vi "DCM DSI Host.vi"() -> ()   [LabVIEW 2016]
uses:
  <vilib>/addons/Software Calibration Management/XControls/SubHost.xctl
  <vilib>/Powertrain Controls/Device Drivers/DCM/Rev0/RT/System State.ctl
  <vilib>/Powertrain Controls/Device Drivers/DCM/Rev0/RT/System ADC.ctl
  <vilib>/Powertrain Controls/Device Drivers/DCM/Rev0/RT/Internal Fault.ctl
  Shared/Typedefs/System-QuickIDsArray.ctl
  <vilib>/addons/Software Calibration Management/xSCM/Controls/ID and Element.ctl
  <vilib>/Utility/miscctls.llb/LVBoundsTypeDef.ctl
  Host/Host SubVIs/VI Ref Global.vi
  <vilib>/Utility/inputDevices.llb/mouseAcquire.vi
  <vilib>/addons/Software Calibration Management/xSCM/SCM-API.lvlib
  <vilib>/Powertrain Controls/Device Drivers/DCM/Rev0/RT/DCM - RT.lvclass
  Shared/DSI-Shared.lvlib
panel:
  in  "_Subhosts":enum32{"Subhosts"}(tab)
  in  "Hidden Settings":T1(xcontrol)={"Name"="System-ExecInfo-Host (System-ExecInfo-Host)", "Host VI"=path "Host/System-ExecInfo-Host.vi", "Pairing File"=path "Host/System-ExecInfo-Host.par", "Display Name"="Execution Information"}
  in  "User Plugin (Engine)":T1(xcontrol)={"Name"="Engine-Throttle-Host (Engine-Throttle-Host)", "Host VI"=path "Host/Engine-Throttle-Host.vi", "Pairing File"=path "Host/Engine-Throttle-Host.par", "Display Name"="Throttle Control Setup"}
  in  "Engine Synchronous TTL Setup":T1(xcontrol)={"Name"="Hardware-DiffIO-Host (Hardware-DiffIO-Host)", "Host VI"=path "Host/Hardware-DiffIO-Host.vi", "Pairing File"=path "Host/Hardware-DiffIO-Host.par", "Display Name"="Differential IO Setup"}
  in  "DI Driver Bank A Setup":T1(xcontrol)={"Name"="Hardware-DI-A-Host (Hardware-DI-A-Host)", "Host VI"=path "Host/Hardware-DI-A-Host.vi", "Pairing File"=path "Host/Hardware-DI-A-Host.par", "Display Name"="DI Driver Bank A Setup"}
  in  "DCM System Setup & State":T1(xcontrol)={"Name"="Hardware-System-Host (Hardware-System-Host)", "Host VI"=path "Host/Hardware-System-Host.vi", "Pairing File"=path "Host/Hardware-System-Host.par", "Display Name"="Hardware System Setup"}
  in  "Half-H Driver Setup":T1(xcontrol)={"Name"="Hardware-HHSetup-Host (Hardware-HHSetup-Host)", "Host VI"=path "Host/Hardware-HHSetup-Host.vi", "Pairing File"=path "Host/Hardware-HHSetup-Host.par", "Display Name"="Half H Setup"}
  in  "DI Driver Bank B Setup":T1(xcontrol)={"Name"="Hardware-DI-B-Host (Hardware-DI-B-Host)", "Host VI"=path "Host/Hardware-DI-B-Host.vi", "Pairing File"=path "Host/Hardware-DI-B-Host.par", "Display Name"="DI Driver Bank B Setup"}
  in  "Differential Digital I/O Setup":T1(xcontrol)={"Name"="Hardware-DiffIO-Host (Hardware-DiffIO-Host)", "Host VI"=path "Host/Hardware-DiffIO-Host.vi", "Pairing File"=path "Host/Hardware-DiffIO-Host.par", "Display Name"="Differential IO Setup"}
  in  "Engine Position Tracking Setup":T1(xcontrol)={"Name"="Hardware-EPTx-Host (Hardware-EPTx-Host)", "Host VI"=path "Host/Hardware-EPTx-Host.vi", "Pairing File"=path "Host/Hardware-EPTx-Host.par", "Display Name"="Engine Position Tracking Setup"}
  in  "CAN Interface":T1(xcontrol)={"Name"="System-CAN-Host (System-CAN-Host)", "Host VI"=path "Host/System-CAN-Host.vi", "Pairing File"=path "Host/System-CAN-Host.par", "Display Name"="CAN Interface"}
  in  "Skip Fire Setup":T1(xcontrol)={"Name"="Hardware-Skipfire-Host (Hardware-Skipfire-Host)", "Host VI"=path "Host/Hardware-Skipfire-Host.vi", "Pairing File"=path "Host/Hardware-Skipfire-Host.par", "Display Name"="Skip Fire Setup"}
  in  "Analog Inputs Setup":T1(xcontrol)={"Name"="Engine-SystemAI-Host (Engine-SystemAI-Host)", "Host VI"=path "Host/Engine-SystemAI-Host.vi", "Pairing File"=path "Host/Engine-SystemAI-Host.par", "Display Name"="Analog Input Setup"}
  in  "DCM System ADC":T1(xcontrol)={"Name"="Hardware-System-Host (Hardware-System-Host)", "Host VI"=path "Host/Hardware-System-Host.vi", "Pairing File"=path "Host/Hardware-System-Host.par", "Display Name"="Hardware System Setup"}
  in  "DI Scope":T1(xcontrol)={"Name"="Engine-DICal-Host (Engine-DICal-Host)", "Host VI"=path "Host/Engine-DICal-Host.vi", "Pairing File"=path "Host/Engine-DICal-Host.par", "Display Name"="Injector Calibration Setup"}
  in  "HH Scope":T1(xcontrol)={"Name"="Engine-Throttle-Host (Engine-Throttle-Host)", "Host VI"=path "Host/Engine-Throttle-Host.vi", "Pairing File"=path "Host/Engine-Throttle-Host.par", "Display Name"="Throttle Control Setup"}
  in  "Plots and Tables":T1(xcontrol)={"Name"="System-ExecInfo-Host (System-ExecInfo-Host)", "Host VI"=path "Host/System-ExecInfo-Host.vi", "Pairing File"=path "Host/System-ExecInfo-Host.par", "Display Name"="Execution Information"}
  in  "Execution Information":T1(xcontrol)={"Name"="System-ExecInfo-Host (System-ExecInfo-Host)", "Host VI"=path "Host/System-ExecInfo-Host.vi", "Pairing File"=path "Host/System-ExecInfo-Host.par", "Display Name"="Execution Information"}
  in  "Channel Data":T1(xcontrol)={"Name"="Engine-SystemAI-Host (Engine-SystemAI-Host)", "Host VI"=path "Host/Engine-SystemAI-Host.vi", "Pairing File"=path "Host/Engine-SystemAI-Host.par", "Display Name"="Analog Input Setup"}
  in  "User Plugin (Asynchronous)":T1(xcontrol)={"Name"="System-User-Host (System-User-Host)", "Host VI"=path "Host/System-User-Host.vi", "Pairing File"=path "Host/System-User-Host.par", "Display Name"="System User VI"}
  in  "DI IPhase Learn":T1(xcontrol)={"Name"="Engine-RPC-Host (Engine-RPC-Host)", "Host VI"=path "Host/Engine-RPC-Host.vi", "Pairing File"=path "Host/Engine-RPC-Host.par", "Display Name"="Rail Pressure Control Setup"}
  in  "DI Control and Calibration":T1(xcontrol)={"Name"="Engine-DICal-Host (Engine-DICal-Host)", "Host VI"=path "Host/Engine-DICal-Host.vi", "Pairing File"=path "Host/Engine-DICal-Host.par", "Display Name"="Injector Calibration Setup"}
  in  "Rail Pressure Control":T1(xcontrol)={"Name"="Engine-RPC-Host (Engine-RPC-Host)", "Host VI"=path "Host/Engine-RPC-Host.vi", "Pairing File"=path "Host/Engine-RPC-Host.par", "Display Name"="Rail Pressure Control Setup"}
  in  "Electronic Throttle Control":T1(xcontrol)={"Name"="Engine-Throttle-Host (Engine-Throttle-Host)", "Host VI"=path "Host/Engine-Throttle-Host.vi", "Pairing File"=path "Host/Engine-Throttle-Host.par", "Display Name"="Throttle Control Setup"}
  in  "User Plugin (Control)":T1(xcontrol)={"Name"="Control-DIFuel-Host (Control-DIFuel-Host)", "Host VI"=path "Host/Control-DIFuel-Host.vi", "Pairing File"=path "Host/Control-DIFuel-Host.par", "Display Name"="DI Fueling Control Setup"}
  in  "Engine Fuel Control":T1(xcontrol)={"Name"="Control-DIFuel-Host (Control-DIFuel-Host)", "Host VI"=path "Host/Control-DIFuel-Host.vi", "Pairing File"=path "Host/Control-DIFuel-Host.par", "Display Name"="DI Fueling Control Setup"}
  out "_DragStart":i32
  in  "UserOS":bool
  out "_IO_Lock":bool caption="I/O Lock"
  out "Sync":bool caption="EPTx"
  in  "SyncEnable":bool
  in  "DI-B_InjectEnable":bool
  in  "DI-A_InjectEnable":bool
  in  "IO_Lock":bool
  in  "MPRD":bool
  in  "SYS|Exec|Password":string
  in  "SYS|Exec|Username":string
  in  "_Help":bool
  out "SYS|Host|Fault":bool
  in  "_AutoFit":bool
  in  "_CalTrend":bool
  in  "_CalScope":bool
  in  "_CalLoad":bool
  in  "_CalSaveAs":bool
  in  "_CalSave":bool
  in  "_RedrawList":bool
  in  "UserOSTime":sgl caption="[s]" format="%#_6p"
  out "_Battery":sgl caption="[V]"
  out "Speed":sgl caption="[RPM]"
  out "_Drive_Power":sgl caption="[V]"
  out "_ConsoleMessages":string caption="SCM Messages"
  in  "_SubHost-List":i32(listbox)=-1
  out "SYS|Exec|CalLoading":bool caption="HW"
  in  "SYS|Plot|Names":string[](array[string])
  out "SYS|Plot|Values":sgl[](array[numeric])
  in  "SYS|Plot|Units":string[](array[string])
  in  "SYS|Plot|IDs":T2
  out "_Subhost-FP.DockStates":bool[](array[boolean])
  out "_Subhost-FP.States":T4(array[ring])=[enum."Closed", enum."Closed", enum."Closed", enum."Closed", enum."Closed", enum."Closed", enum."Closed", enum."Closed", enum."Closed", enum."Closed", enum."Closed", enum."Closed", enum."Closed", enum."Closed", enum."Closed", enum."Closed", enum."Closed", enum."Closed", enum."Closed"]
  in  "_QuickValues":i32(listbox) caption="Quick Values"
  in  "SYS|Plot|Select":u8
  out "State":T5 {"System ADC"."Fan [V]" format="%#_3p"; "System ADC"."Primary B1B2 [V]" format="%#_3p"; "System ADC"."Primary B3B4 [V]" format="%#_3p"; "System ADC"."Primary A3A4 [V]" format="%#_3p"; "System ADC"."Primary A1A2 [V]" format="%#_3p"; "System ADC"."MPRD [V]" format="%#_3p"; "System ADC"."Ext HV B [V]" format="%#_3p"; "System ADC"."Ext HV A [V]" format="%#_3p"; "System ADC"."Pump Zener B [V]" format="%#_3p"; "System ADC"."Pump Zener A [V]" format="%#_3p"; "System ADC"."DI Zener B [V]" format="%#_3p"; "System ADC"."DI Zener A [V]" format="%#_3p"; "System ADC"."Key [V]" format="%#_3p"; "System ADC"."DRVP [V]" format="%#_3p"; "System ADC"."Battery [V]" format="%#_3p"; "System ADC"."FET Driver [V]" format="%#_3p"; "System ADC"."Secondary B1B2 [V]" format="%#_3p"; "System ADC"."Secondary B3B4 [V]" format="%#_3p"; "System ADC"."Secondary A3A4 [V]" format="%#_3p"; "System ADC"."Secondary A1A2 [V]" format="%#_3p"; "System ADC"."Primary Range [V]" format="%#_3p"; "System ADC"."Temp Boost B [C]" format="%#_3p"; "System ADC"."Temp Primary A [C]" format="%#_3p"; "System ADC"."Temp Secondary A [C]" format="%#_3p"; "System ADC"."Temp Fan Intake [C]" format="%#_3p"; "System ADC"."Temp CPU [C]" format="%#_3p"; "System ADC"."Temp DI Zener B [C]" format="%#_3p"; "System ADC"."Temp DI B [C]" format="%#_3p"; "System ADC"."Temp DI Zener A [C]" format="%#_3p"; "System ADC"."Temp DI A [C]" format="%#_3p"; "System ADC"."Temp HH 7-12 [C]" format="%#_3p"; "System ADC"."Temp HH 1-6 [C]" format="%#_3p"; "System ADC"."AI 12 [V]" format="%#_3p"; "System ADC"."AI 11 [V]" format="%#_3p"; "System ADC"."AI 10 [V]" format="%#_3p"; "System ADC"."AI 9 [V]" format="%#_3p"; "System ADC"."AI 8 [V]" format="%#_3p"; "System ADC"."AI 7 [V]" format="%#_3p"; "System ADC"."AI 6 [V]" format="%#_3p"; "System ADC"."AI 5 [V]" format="%#_3p"; "System ADC"."AI 4 [V]" format="%#_3p"; "System ADC"."AI 3 [V]" format="%#_3p"; "System ADC"."AI 2 [V]" format="%#_3p"; "System ADC"."AI 1 [V]" format="%#_3p"}
  # "Password"
  # "Username"
  # "One-Shot Time"
  # "Batt"
  # "Speed"
  # "DRVP"
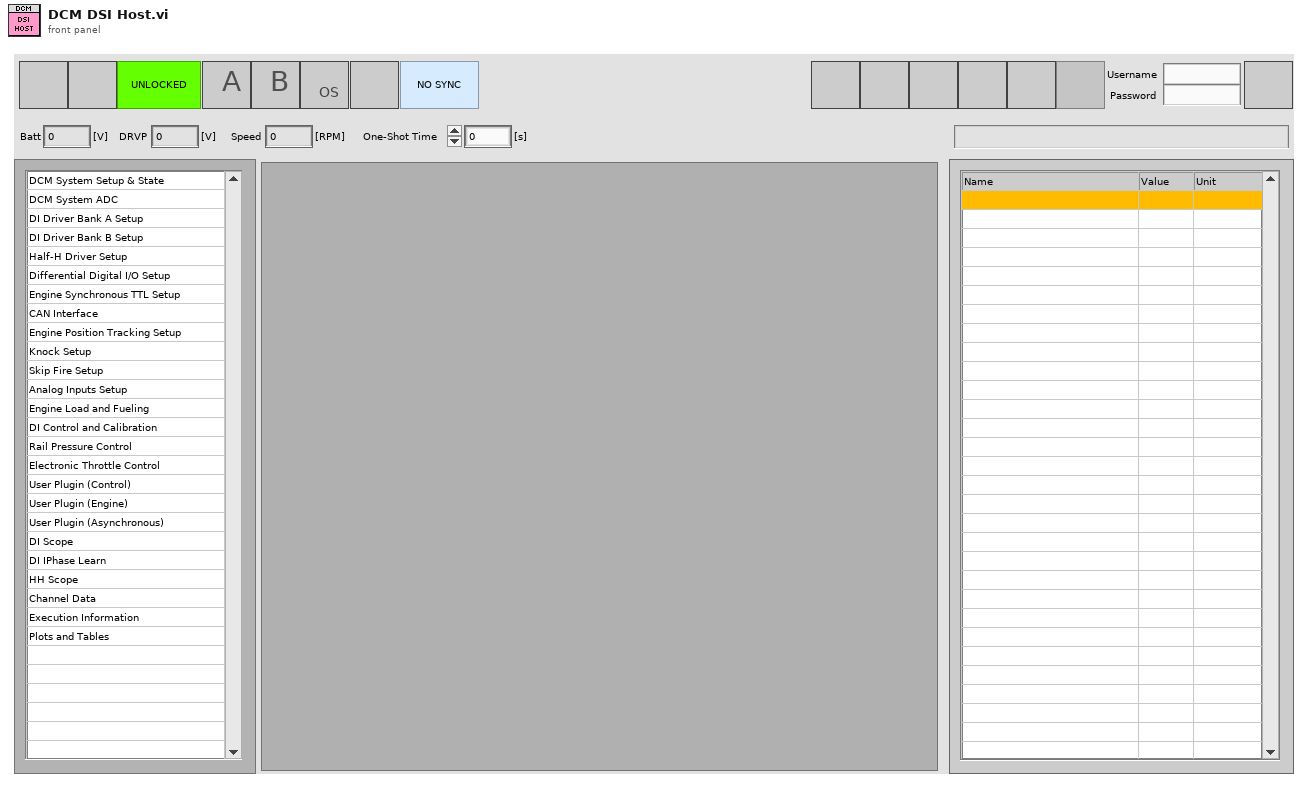
[diagram p1: front panel]
types:
  T1 = cluster{"Name":string, "Host VI":path, "Pairing File":path, "Display Name":string}
  T2 = typedef "DSI-Shared.lvlib/System-QuickIDsArray.ctl" = T3[]
  T3 = typedef "SCM-API.lvlib/ID and Element.ctl" = cluster{"ID":u32, "Element":i32[]}
  T4 = enum32{"Invalid", "Standard", "Closed", "Hidden", "Minimized", "Maximized"}[]
  T5 = typedef "DCM - RT.lvclass/System State.ctl" = cluster{"System ADC":T6, "IO Lock":bool, "HH Mode Config Error":bool, "Fan Speed 1 [RPM]":sgl, "Fan Speed 2 [RPM]":sgl, "Firmware Major Rev":u16, "Firmware Minor Rev":u16, "Internal Fault":T7, "Fault Value":dbl}
  T6 = typedef "DCM - RT.lvclass/System ADC.ctl" = cluster{"AI 1 [V]":sgl, "AI 2 [V]":sgl, "AI 3 [V]":sgl, "AI 4 [V]":sgl, "AI 5 [V]":sgl, "AI 6 [V]":sgl, "AI 7 [V]":sgl, "AI 8 [V]":sgl, "AI 9 [V]":sgl, "AI 10 [V]":sgl, "AI 11 [V]":sgl, "AI 12 [V]":sgl, "Temp HH 1-6 [C]":sgl, "Temp HH 7-12 [C]":sgl, "Temp DI A [C]":sgl, "Temp DI Zener A [C]":sgl, "Temp DI B [C]":sgl, "Temp DI Zener B [C]":sgl, "Temp CPU [C]":sgl, "Temp Fan Intake [C]":sgl, "Temp Secondary A [C]":sgl, "Temp Primary A [C]":sgl, "Temp Boost B [C]":sgl, "Primary Range [V]":sgl, "Primary A1A2 [V]":sgl, "Primary A3A4 [V]":sgl, "Primary B3B4 [V]":sgl, "Primary B1B2 [V]":sgl, "Secondary A1A2 [V]":sgl, "Secondary A3A4 [V]":sgl, "Secondary B3B4 [V]":sgl, "Secondary B1B2 [V]":sgl, "Ext HV A [V]":sgl, "Ext HV B [V]":sgl, "FET Driver [V]":sgl, "Fan [V]":sgl, "Battery [V]":sgl, "DRVP [V]":sgl, "Key [V]":sgl, "DI Zener A [V]":sgl, "DI Zener B [V]":sgl, "Pump Zener A [V]":sgl, "Pump Zener B [V]":sgl, "MPRD [V]":sgl}
  T7 = typedef "DCM - RT.lvclass/Internal Fault.ctl" = enum32{"None", "Temp HH 1-6", "Temp HH 7-12", "Temp DI A", "Temp DI Zener A", "Temp DI B", "Temp DI Zener B", "Temp Intake", "Temp Primary A", "Temp Secondary A", "Temp Boost B", "Temp CPU", "Low Battery", "Inrush Protection", "A Run Enable", "B Run Enable", "Fan Speed"}
  T8 = typedef "LVBoundsTypeDef.ctl" = cluster{"Width":u32, "Height":u32}
  T9 = enum8{"Enabled", "Disabled", "Disabled and Grayed Out"}
  T10 = enum32{"Invalid", "Standard", "Closed", "Hidden", "Minimized", "Maximized"}
  T11 = enum16{"Save Workspace", "Exit", "Stop Host Application", "Stop Target", "Set Target Time", "Fault File", "Fault Display", "Silence Alarms", "Calibration Differencer", "Save Calibration", "Save Calibration As", "Get Calibration File", "Set Calibration File", "Load Calibration File", "CalScope", "CalTrend"}
  T12 = cluster{u32, "DCM System Setup & State":cluster{"Name":string, "Host VI":path, "Pairing File":path, "Display Name":string}}
  T13 = cluster{u32, "DCM System ADC":cluster{"Name":string, "Host VI":path, "Pairing File":path, "Display Name":string}}
  T14 = cluster{u32, "DI Driver Bank A Setup":cluster{"Name":string, "Host VI":path, "Pairing File":path, "Display Name":string}}
  T15 = cluster{u32, "DI Driver Bank B Setup":cluster{"Name":string, "Host VI":path, "Pairing File":path, "Display Name":string}}
  T16 = cluster{u32, "Half-H Driver Setup":cluster{"Name":string, "Host VI":path, "Pairing File":path, "Display Name":string}}
  T17 = cluster{u32, "Differential Digital I/O Setup":cluster{"Name":string, "Host VI":path, "Pairing File":path, "Display Name":string}}
  T18 = cluster{u32, "Engine Synchronous TTL Setup":cluster{"Name":string, "Host VI":path, "Pairing File":path, "Display Name":string}}
  T19 = cluster{u32, "CAN Interface":cluster{"Name":string, "Host VI":path, "Pairing File":path, "Display Name":string}}
  T20 = cluster{u32, "Engine Position Tracking Setup":cluster{"Name":string, "Host VI":path, "Pairing File":path, "Display Name":string}}
  T21 = cluster{u32, "Skip Fire Setup":cluster{"Name":string, "Host VI":path, "Pairing File":path, "Display Name":string}}
  T22 = cluster{u32, "Analog Inputs Setup":cluster{"Name":string, "Host VI":path, "Pairing File":path, "Display Name":string}}
  T23 = cluster{u32, "Engine Fuel Control":cluster{"Name":string, "Host VI":path, "Pairing File":path, "Display Name":string}}
  T24 = cluster{u32, "DI Control and Calibration":cluster{"Name":string, "Host VI":path, "Pairing File":path, "Display Name":string}}
  T25 = cluster{u32, "Rail Pressure Control":cluster{"Name":string, "Host VI":path, "Pairing File":path, "Display Name":string}}
  T26 = cluster{u32, "Electronic Throttle Control":cluster{"Name":string, "Host VI":path, "Pairing File":path, "Display Name":string}}
  T27 = cluster{u32, "User Plugin (Control)":cluster{"Name":string, "Host VI":path, "Pairing File":path, "Display Name":string}}
  T28 = cluster{u32, "User Plugin (Engine)":cluster{"Name":string, "Host VI":path, "Pairing File":path, "Display Name":string}}
  T29 = cluster{u32, "DI Scope":cluster{"Name":string, "Host VI":path, "Pairing File":path, "Display Name":string}}
  T30 = cluster{u32, "DI IPhase Learn":cluster{"Name":string, "Host VI":path, "Pairing File":path, "Display Name":string}}
  T31 = cluster{u32, "HH Scope":cluster{"Name":string, "Host VI":path, "Pairing File":path, "Display Name":string}}
  T32 = cluster{u32, "Channel Data":cluster{"Name":string, "Host VI":path, "Pairing File":path, "Display Name":string}}
  T33 = cluster{u32, "Execution Information":cluster{"Name":string, "Host VI":path, "Pairing File":path, "Display Name":string}}
  T34 = cluster{u32, "Plots and Tables":cluster{"Name":string, "Host VI":path, "Pairing File":path, "Display Name":string}}
  T35 = cluster{u32, "User Plugin (Asynchronous)":cluster{"Name":string, "Host VI":path, "Pairing File":path, "Display Name":string}}
  T36 = cluster{u32, "Plots and Tables":cluster{"Name":string, "Host VI":path, "Pairing File":path, "Display Name":string}}[]
  T37 = cluster{"button 1":bool, "button 2":bool, "button 3":bool, "button 4":bool}
  T38 = cluster{"Shift":bool, "Ctrl":bool, "Alt":bool, "Cmd":bool, "Opt":bool}
  T39 = typedef "eventvkey.ctl" = enum16{"ASCII", "Enter", "Return", "Shift", "Ctrl", "Alt", "Cmd", "Opt", "Caps", "NumLock", "Clear", "Break", "Up", "Down", "Left", "Right", "Insert", "Delete", "Home", "End", "PageUp", "PageDown", "Escape", "Help", "Pause", "ScrollLock", "F1", "F2", "F3", "F4", "F5", "F6", "F7", "F8", "F9", "F10", "F11", "F12", "F13", "F14", "F15", "F16", "F17", "F18", "F19", "F20", "F21", "F22", "F23", "F24", "Play", "VolumeUp", "VolumeDown", "Mute", "Two Byte Char"}
  T40 = typedef "LVPointTypeDef.ctl" = cluster{"Horizontal":i16, "Vertical":i16}
  T41 = enum16{"Always On", "Always Off", "Off While Running"}
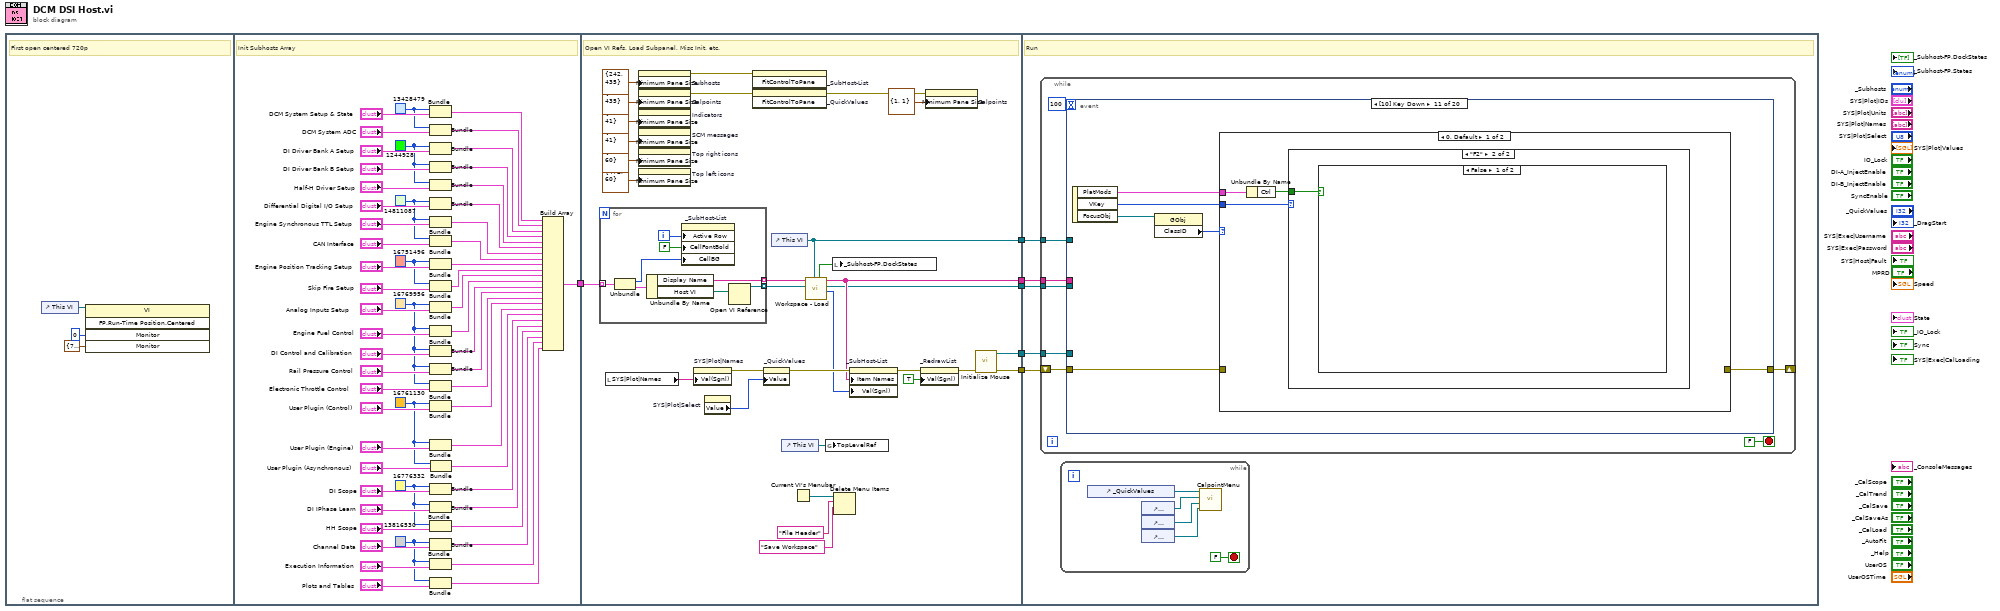
[diagram p0: block diagram]
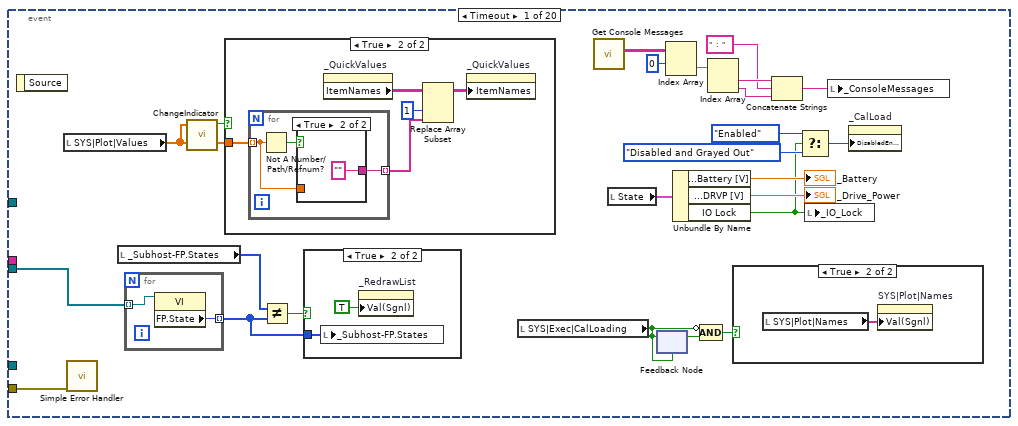
[diagram p2: hidden frame]
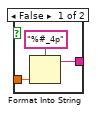
[diagram p4: hidden frame]
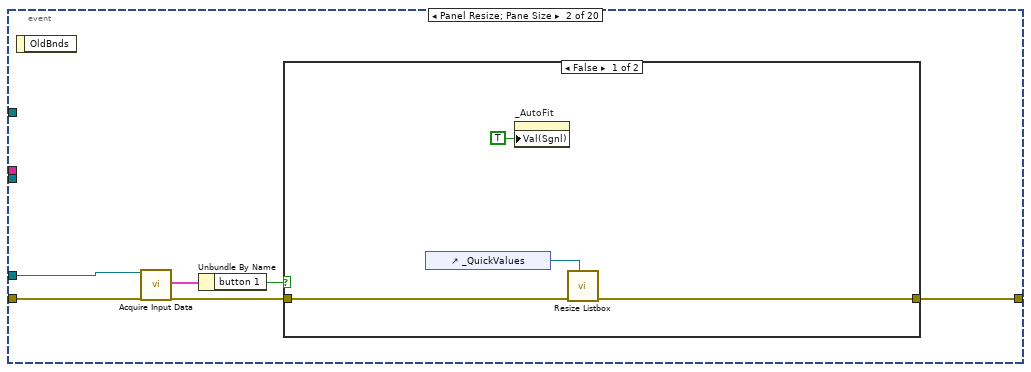
[diagram p7: hidden frame]
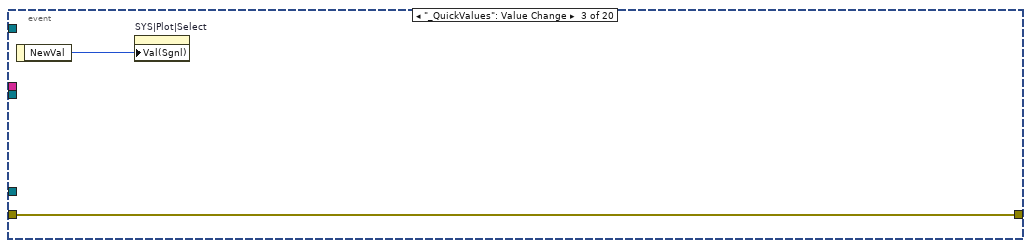
[diagram p9: hidden frame]
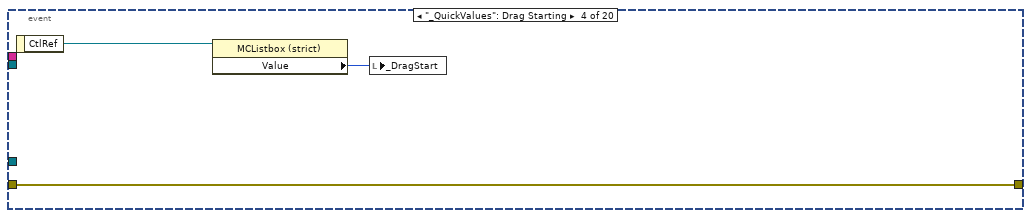
[diagram p10: hidden frame]
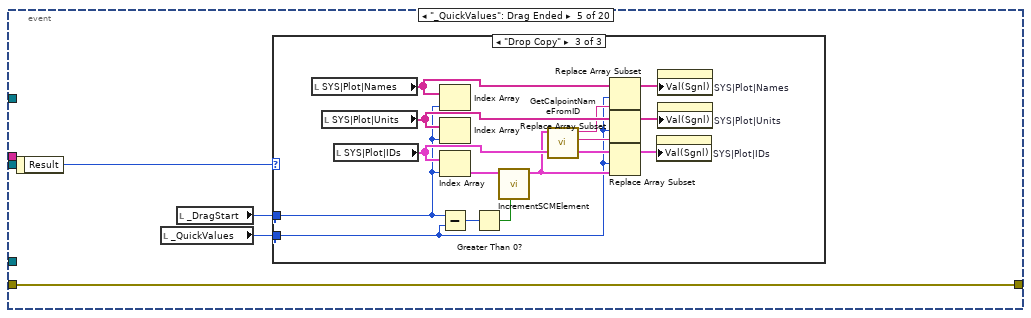
[diagram p11: hidden frame]
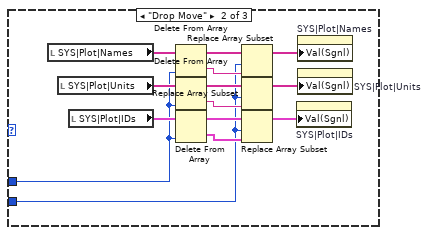
[diagram p13: hidden frame]
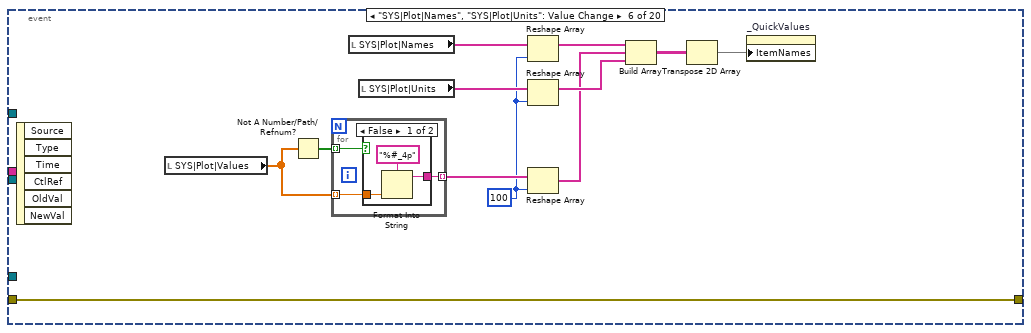
[diagram p14: hidden frame]
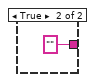
[diagram p15: hidden frame]
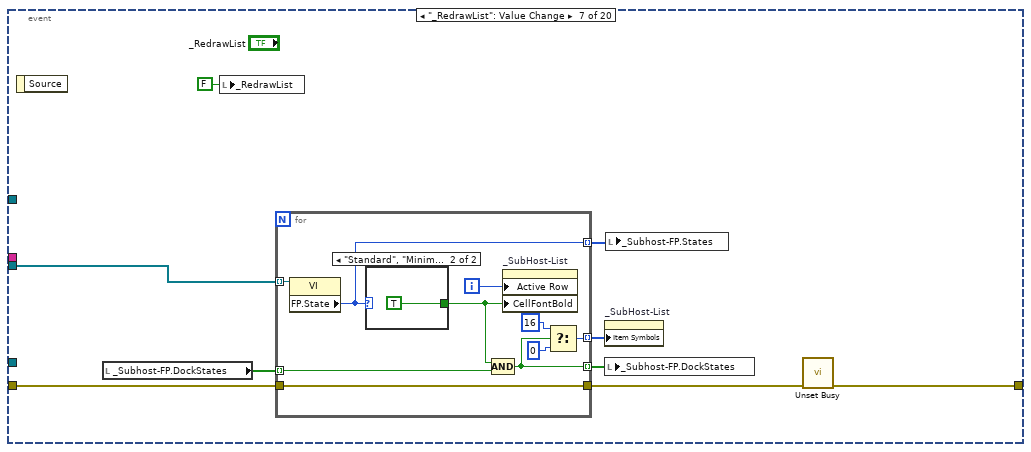
[diagram p16: hidden frame]
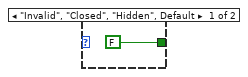
[diagram p17: hidden frame]
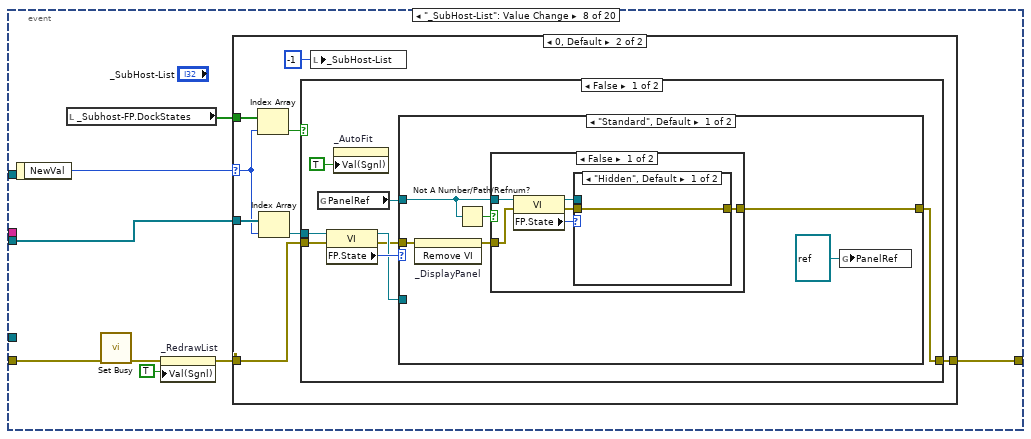
[diagram p18: hidden frame]
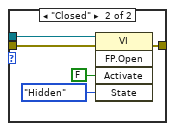
[diagram p20: hidden frame]
diagram:
  n1 = flat-sequence {
    tunnel: [w40] -> w6
    tunnel: w6 -> [w80]
    tunnel: [w68] -> w5
    tunnel: [w93] -> w4
    tunnel: [w79] -> w3
    tunnel: [w83] -> w2
    tunnel: [w73] -> w1
    tunnel: w5 -> [w110]
    tunnel: w4 -> [w109]
    tunnel: w3 -> [w108]
    tunnel: w2 -> [w107]
    tunnel: w1 -> [w106]
    frame #0 {
      # "First open centered 720p"
      n2 = control-ref of="This VI"() -> (w9:refnum<vi>)
      n3 = invoke class="VI" method="FP.Run-Time Position.Centered"(reference=w9, "Monitor"=i16 0, "Monitor"=cluster{"Height":i16, "Width":i16} {"Height"=720, "Width"=1280} ("Size")) -> ()  [unwired: 2 in, 5 out]
    }
    frame #1 {
      w14 = u32 16776332
      w10 = u32 16761130
      w15 = u32 16769956
      w16 = u32 16751496
      w17 = u32 1244928
      w18 = u32 14811087
      w27 = u32 13816530
      w28 = u32 13428479
      # "Init Subhosts Array"
      n4 = Bundle(w28, "DCM System Setup & State"="DCM System Setup & State") -> (w63:T12)  [unwired: 1 in]
      n5 = Bundle(w28, "DCM System ADC"="DCM System ADC") -> (w64:T13)  [unwired: 1 in]
      n6 = Bundle(w17, "DI Driver Bank A Setup"="DI Driver Bank A Setup") -> (w46:T14)  [unwired: 1 in]
      n7 = Bundle(w17, "DI Driver Bank B Setup"="DI Driver Bank B Setup") -> (w47:T15)  [unwired: 1 in]
      n8 = Bundle(w17, "Half-H Driver Setup"="Half-H Driver Setup") -> (w48:T16)  [unwired: 1 in]
      n9 = Bundle(w18, "Differential Digital I/O Setup"="Differential Digital I/O Setup") -> (w49:T17)  [unwired: 1 in]
      n10 = Bundle(w18, "Engine Synchronous TTL Setup"="Engine Synchronous TTL Setup") -> (w30:T18)  [unwired: 1 in]
      n11 = Bundle(w18, "CAN Interface"="CAN Interface") -> (w33:T19)  [unwired: 1 in]
      n12 = Bundle(w16, "Engine Position Tracking Setup"="Engine Position Tracking Setup") -> (w50:T20)  [unwired: 1 in]
      n13 = Bundle(w16, "Skip Fire Setup"="Skip Fire Setup") -> (w57:T21)  [unwired: 1 in]
      n14 = Bundle(w15, "Analog Inputs Setup"="Analog Inputs Setup") -> (w54:T22)  [unwired: 1 in]
      n15 = Bundle(w15, "Engine Fuel Control"="Engine Fuel Control") -> (w61:T23)  [unwired: 1 in]
      n16 = Bundle(w15, "DI Control and Calibration"="DI Control and Calibration") -> (w22:T24)  [unwired: 1 in]
      n17 = Bundle(w15, "Rail Pressure Control"="Rail Pressure Control") -> (w21:T25)  [unwired: 1 in]
      n18 = Bundle(w15, "Electronic Throttle Control"="Electronic Throttle Control") -> (w20:T26)  [unwired: 1 in]
      n19 = Bundle(w10, "User Plugin (Control)"="User Plugin (Control)") -> (w19:T27)  [unwired: 1 in]
      n20 = Bundle(w10, "User Plugin (Engine)"="User Plugin (Engine)") -> (w23:T28)  [unwired: 1 in]
      n21 = Bundle(w14, "DI Scope"="DI Scope") -> (w24:T29)  [unwired: 1 in]
      n22 = Bundle(w14, "DI IPhase Learn"="DI IPhase Learn") -> (w25:T30)  [unwired: 1 in]
      n23 = Bundle(w14, "HH Scope"="HH Scope") -> (w26:T31)  [unwired: 1 in]
      n24 = Bundle(w27, "Channel Data"="Channel Data") -> (w37:T32)  [unwired: 1 in]
      n25 = Bundle(w27, "Execution Information"="Execution Information") -> (w38:T33)  [unwired: 1 in]
      n26 = Bundle(w27, "Plots and Tables"="Plots and Tables") -> (w39:T34)  [unwired: 1 in]
      n27 = Bundle(w10, "User Plugin (Asynchronous)"="User Plugin (Asynchronous)") -> (w13:T35)  [unwired: 1 in]
      n28 = Build Array(w63, w64, w46, w47, w48, w49, w30, w33, w50, w57, w54, w61, w22, w21, w20, w19, w23, w13, w24, w25, w26, w37, w38, w39) -> (w40:T36)
    }
    frame #2 {
      # "Open VI Refs, Load Subpanel, Misc Init, etc."
      n29 = for {
        tunnel: w80 -> [w104] mode=indexing
        tunnel: [w101] -> w78 mode=indexing
        tunnel: [w98] -> w77 mode=indexing
        i -> [w103]
        n30 = Unbundle(w104) -> (w100:u32, "Plots and Tables"=w105:T1)
        n31 = Unbundle By Name(w105) -> ("Display Name"=w101:string, "Host VI"=w99:path)
        n32 = property on="_SubHost-List" class="LstBox (strict)"("Active Row"=w103, "CellFontBold"=FALSE ("Active Row:Cell Font:Bold"), "CellBG"=w100) -> ()  [unwired: 2 in, 2 out]
        n33 = Open VI Reference(vi path=w99) -> (vi reference=w98:refnum<vi>)  [unwired: 5 in, 1 out]
      }
      n34 = local read "SYS|Plot|Names"() -> (w97:string[])
      n35 = property on="Subhosts" class="Pane"("Minimum Pane Size"=T8 {"Width"=242, "Height"=435} ("Bounds 1")) -> (error out=w71:errorcluster)  [unwired: 2 in, 1 out]
      n36 = property on="Calpoints" class="Pane"("Minimum Pane Size"=T8 {"Width"=346, "Height"=435} ("Bounds 2")) -> (error out=w72:errorcluster)  [unwired: 2 in, 1 out]
      n37 = property on="Indicators" class="Pane"("Minimum Pane Size"=T8 {"Width"=607, "Height"=41} ("Bounds 3")) -> ()  [unwired: 2 in, 2 out]
      n38 = property on="SCM messages" class="Pane"("Minimum Pane Size"=T8 {"Width"=345, "Height"=41} ("Bounds 4")) -> ()  [unwired: 2 in, 2 out]
      n39 = property on="Top right icons" class="Pane"("Minimum Pane Size"=T8 {"Width"=486, "Height"=60} ("Bounds 5")) -> ()  [unwired: 2 in, 2 out]
      n40 = property on="Top left icons" class="Pane"("Minimum Pane Size"=T8 {"Width"=472, "Height"=60} ("Bounds 6")) -> ()  [unwired: 2 in, 2 out]
      n41 = property on="SYS|Plot|Names" class="Arr (strict)"("Val(Sgnl)"=w97) -> (error out=w96:errorcluster)  [unwired: 2 in, 1 out]
      n42 = property on="SYS|Plot|Select" class="DigNum (strict)"() -> ("Value"=w94:u8)  [unwired: 2 in, 2 out]
      n43 = invoke on="_SubHost-List" class="LstBox (strict)" method="FitControlToPane"(error in=w71) -> ()  [unwired: 2 in, 3 out]
      n44 = invoke on="_QuickValues" class="MCListbox (strict)" method="FitControlToPane"(error in=w72) -> (error out=w69:errorcluster)  [unwired: 2 in, 2 out]
      n45 = property on="_QuickValues" class="MCListbox (strict)"(error in=w96, "Value"=w94) -> (error out=w95:errorcluster)  [unwired: 1 in, 1 out]
      n46 = control-ref of="This VI"() -> (w73:refnum<vi>)
      n47 = control-ref of="This VI"() -> (w67:refnum<vi>)
      n48 = Current VI's Menubar() -> (w76:refnum<k9>)
      n49 = call "Workspace - Load.vi"("This VI"=w73, "VI Refs"=w77, "Subhost Names"=w78) -> ("PanelSubhost"=w82:i32, "VI Refs out"=w68:refnum<vi>[], "Subhost Names out"=w79:string[], "_Subhost-FP.DockStates"=w81:bool[])  [unwired: 4 in, 1 out]
      n50 = global write "VI Ref Global.vi" "TopLevelRef"(w67) -> ()
      n51 = local write "_Subhost-FP.DockStates"(w81) -> ()
      n52 = Delete Menu Items(7:"Save Workspace" ("items"), 8:"File Header" ("item tag"), 9:w76) -> ()  [unwired: 1 in, 2 out]
      n53 = property on="_SubHost-List" class="LstBox (strict)"(error in=w95, "Item Names"=w79, "Val(Sgnl)"=w82) -> (error out=w91:errorcluster)  [unwired: 1 in, 1 out]
      n54 = property on="_RedrawList" class="Bool (strict)"(error in=w91, "Val(Sgnl)"=TRUE ("Value (Signaling)")) -> (error out=w90:errorcluster)  [unwired: 1 in, 1 out]
      n55 = property on="Calpoints" class="Pane"(error in=w69, "Minimum Pane Size"=T8 {"Width"=1, "Height"=1} ("Bounds 2")) -> ()  [unwired: 1 in, 2 out]
      n56 = call <vilib>:"Initialize Mouse.vi"("error in (no error)"=w90) -> ("error out"=w83:errorcluster, "device ID"=w93:refnum<k1>)  [unwired: 9 in]
    }
    frame #3 {
      # "Run"
      n57 = while {
        tunnel: w110 -> [w122]
        shift-right: [w116] -> _
        shift-left: w107 -> [w117]
        tunnel: w109 -> [w121]
        tunnel: w106 -> [w120]
        tunnel: w108 -> [w119]
        stop <- FALSE ("status") stop-if-true
        n58 = event shown="[10] Key Down" {
          selector: _ -> [_ _ _ _ _ _ _ _ _ _ _ _ _ _ _ _ _ _ _ _]
          dyn-events: _ -> [_ _ _ _ _ _ _ _ _ _ _ _ _ _ _ _ _ _ _ _]
          timeout: 100 -> [_ _ _ _ _ _ _ _ _ _ _ _ _ _ _ _ _ _ _ _]
          tunnel: w122 -> [w147 _ _ _ _ _ w240 w258 w334 w370 _ _ _ _ _ _ _ _ _ w556]
          tunnel: w117 -> [w133 w167 w176 w178 w181 w213 w233 w255 w336 w365 w435 w463 w465 w468 w471 w474 w477 w484 w549 _]
          tunnel: [_ w165 w176 w178 w181 w213 w234 w254 w335 w367 w436 w463 w465 w468 w471 w474 w477 w483 w549 _] -> w116
          tunnel: w121 -> [_ w170 _ _ _ _ _ _ _ _ _ _ _ _ _ _ _ _ _ _]
          tunnel: w120 -> [_ _ _ _ _ _ _ _ _ _ _ _ _ _ _ _ _ w480 _ w554]
          tunnel: w119 -> [_ _ _ _ _ _ _ _ _ _ _ _ _ _ _ _ _ _ _ w557]
          event Timeout {
            n59 = event-data() -> ()  [unwired: 1 in, 1 out]
            n60 = local read "SYS|Plot|Values"() -> (w124:sgl[])
            n61 = call <vilib>:"Simple Error Handler.vi"("error in (no error)"=w133) -> ()  [unwired: 4 in, 5 out]
            n62 = local read "_Subhost-FP.States"() -> (w146:T4)
            n63 = for {
              tunnel: w147 -> [w164] mode=indexing
              tunnel: [w163] -> w144 mode=indexing
              n64 = property class="VI"(reference=w164) -> ("FP.State"=w163:T10)  [unwired: 1 in, 2 out]
            }
            n65 = call "ChangeIndicator.vi"("Input"=w124) -> ("Change"=w125:bool)  [unwired: 9 in]
            n66 = case shown="True" w125 {
              tunnel: w124 -> [_ w152]
              frame False {
              }
              frame True {
                n67 = for {
                  tunnel: w152 -> [w154] mode=indexing
                  tunnel: [w155] -> w151 mode=indexing
                  n68 = Not A Number/Path/Refnum?(number/path/refnum=w154) -> (NaN/Path/Refnum?=w153:bool)
                  n69 = case shown="True" w153 {
                    tunnel: w154 -> [w157 _]
                    tunnel: [w158 ""] -> w155
                    frame False {
                      n70 = Format Into String(format string="%#_4p", w157) -> (resulting string=w158:string)  [unwired: 2 in, 1 out]
                    }
                    frame True {
                    }
                  }
                }
                n71 = property on="_QuickValues" class="MCListbox (strict)"() -> ("ItemNames"=w148:string[][])  [unwired: 2 in, 2 out]
                n72 = Replace Array Subset(array=w148, new element=w151, index (col)=1 ("disabled index (col)")) -> (w149:string[][])  [unwired: 1 in]
                n73 = property on="_QuickValues" class="MCListbox (strict)"("ItemNames"=w149) -> ()  [unwired: 2 in, 2 out]
              }
            }
            n74 = Not Equal?(x=w146, y=w144) -> (x != y?=w145:bool)
            n75 = case shown="True" w145 {
              tunnel: w144 -> [_ w161]
              frame False {
              }
              frame True {
                n76 = local write "_Subhost-FP.States"(w161) -> ()
                n77 = property on="_RedrawList" class="Bool (strict)"("Val(Sgnl)"=TRUE ("Value (Signaling)")) -> ()  [unwired: 2 in, 2 out]
              }
            }
            n78 = local read "SYS|Exec|CalLoading"() -> (w140:bool)
            n79 = call <vilib>:"Get Console Messages.vi"() -> ("Messages"=w131:string[][])  [unwired: 10 in, 1 out]
            n80 = local read "State"() -> (w143:T5)
            n81 = feedback #1(w140) -> (w142:bool)
            n82 = feedback-in #1(w140) -> ()
            n83 = Index Array(array=w131, index (row)=0) -> (element=w130:string[])  [unwired: 1 in]
            n84 = Unbundle By Name(w143) -> ("System ADC.Battery [V]"=→"_Battery":sgl, "System ADC.DRVP [V]"=→"_Drive_Power":sgl, "IO Lock"=w134:bool)
            n85 = Compound Arithmetic op=AND(invert w140, w142) -> (w141:bool)
            n86 = Index Array(array=w130) -> (element #1=w129:string, element #2=w128:string)  [unwired: 2 in]
            n87 = case shown="True" w141 {
              frame False {
              }
              frame True {
                n88 = local read "SYS|Plot|Names"() -> (w160:string[])
                n89 = property on="SYS|Plot|Names" class="Arr (strict)"("Val(Sgnl)"=w160) -> ()  [unwired: 2 in, 2 out]
              }
            }
            n90 = Concatenate Strings(w129, "  :  " ("string"), w128) -> (w126:string)
            n91 = Select(t=T9."Enabled" ("Disabled"), s=w134, f=T9."Disabled and Grayed Out" ("Disabled")) -> (s? t:f=w137:T9)
            n92 = local write "_IO_Lock"(w134) -> ()
            n93 = local write "_ConsoleMessages"(w126) -> ()
            n94 = property on="_CalLoad" class="Bool (strict)"("DisabledEnum"=w137) -> ()  [unwired: 2 in, 2 out]
          }
          event Panel Resize; Pane Size {
            n95 = event-data() -> ()  [unwired: 1 in, 1 out]
            n96 = call-poly <vilib>:"Acquire Input Data.vi"("device ID"=w170, "error in (no error)"=w167) -> ("button info"=w169:T37, "error out"=w166:errorcluster)  [unwired: 14 in, 2 out]
            n97 = Unbundle By Name(w169) -> ("button 1"=w168:bool)
            n98 = case shown="False" w168 {
              tunnel: w166 -> [w173 w175]
              tunnel: [w171 w175] -> w165
              frame False {
                n99 = control-ref of="_QuickValues"() -> (w172:refnum<vi>)
                n100 = property on="_AutoFit" class="Bool (strict)"("Val(Sgnl)"=TRUE ("Value (Signaling)")) -> ()  [unwired: 2 in, 2 out]
                n101 = call "Resize Listbox.vi"("MulticolumnListbox in"=w172, "error in (no error)"=w173) -> ("error out"=w171:errorcluster)  [unwired: 9 in]
              }
              frame True {
              }
            }
          }
          event "_QuickValues": Value Change {
            n102 = event-data() -> ("NewVal"=w177:i32)  [unwired: 1 in]
            n103 = property on="SYS|Plot|Select" class="DigNum (strict)"("Val(Sgnl)"=w177) -> ()  [unwired: 2 in, 2 out]
          }
          event "_QuickValues": Drag Starting {
            n104 = event-data() -> ("CtlRef"=w180:refnum<vi>)  [unwired: 1 in]
            n105 = property class="MCListbox (strict)"(reference=w180) -> ("Value"=w179:i32)  [unwired: 1 in, 2 out]
            n106 = local write "_DragStart"(w179) -> ()
          }
          event "_QuickValues": Drag Ended {
            n107 = event-data() -> ("Result"=w184:enum16{"Drop Cancel", "Drop Move", "Drop Copy"})  [unwired: 1 in]
            n108 = local read "_QuickValues"() -> (w182:i32)
            n109 = local read "_DragStart"() -> (w183:i32)
            n110 = case shown="\"Drop Copy\"" w184 {
              tunnel: w183 -> [_ w186 w202]
              tunnel: w182 -> [_ w185 w201]
              frame "Drop Cancel", Default {
              }
              frame "Drop Move" {
                n111 = local read "SYS|Plot|Names"() -> (w198:string[])
                n112 = local read "SYS|Plot|Units"() -> (w195:string[])
                n113 = local read "SYS|Plot|IDs"() -> (w194:T2)
                n114 = Delete From Array(array=w198, index=w186) -> (deleted portion=w189:string, array with subset deleted=w197:string[])  [unwired: 1 in]
                n115 = Delete From Array(array=w195, index=w186) -> (deleted portion=w188:string, array with subset deleted=w196:string[])  [unwired: 1 in]
                n116 = Delete From Array(array=w194, index=w186) -> (deleted portion=w187:T3, array with subset deleted=w193:T2)  [unwired: 1 in]
                n117 = Replace Array Subset(array=w197, new element=w189, index=w185) -> (w192:string[])
                n118 = Replace Array Subset(array=w196, new element=w188, index=w185) -> (w191:string[])
                n119 = Replace Array Subset(array=w193, new element=w187, index=w185) -> (w190:T2)
                n120 = property on="SYS|Plot|IDs" class="Arr (strict)"("Val(Sgnl)"=w190) -> ()  [unwired: 2 in, 2 out]
                n121 = property on="SYS|Plot|Names" class="Arr (strict)"("Val(Sgnl)"=w192) -> ()  [unwired: 2 in, 2 out]
                n122 = property on="SYS|Plot|Units" class="Arr (strict)"("Val(Sgnl)"=w191) -> ()  [unwired: 2 in, 2 out]
              }
              frame "Drop Copy" {
                n123 = local read "SYS|Plot|Names"() -> (w207:string[])
                n124 = local read "SYS|Plot|Units"() -> (w208:string[])
                n125 = local read "SYS|Plot|IDs"() -> (w209:T2)
                n126 = Index Array(array=w207, index=w202) -> ()  [unwired: 1 out]
                n127 = Index Array(array=w208, index=w202) -> ()  [unwired: 1 out]
                n128 = Index Array(array=w209, index=w202) -> (element=w206:T3)
                n129 = Subtract(x=w202, y=w201) -> (x-y=w200:i32)
                n130 = Greater Than 0?(x=w200) -> (x > 0?=w199:bool)
                n131 = call "IncrementSCMElement.vi"("Decrement? (F)"=w199, "ID in"=w206) -> ("ID out"=w205:T3)  [unwired: 9 in]
                n132 = call "GetCalpointNameFromID.vi"("ID"=w205) -> ("Units"=w203:string, "Name"=w204:string)  [unwired: 9 in]
                n133 = Replace Array Subset(array=w207, new element=w204, index=w201) -> (w212:string[])
                n134 = Replace Array Subset(array=w208, new element=w203, index=w201) -> (w211:string[])
                n135 = Replace Array Subset(array=w209, new element=w205, index=w201) -> (w210:T2)
                n136 = property on="SYS|Plot|IDs" class="Arr (strict)"("Val(Sgnl)"=w210) -> ()  [unwired: 2 in, 2 out]
                n137 = property on="SYS|Plot|Names" class="Arr (strict)"("Val(Sgnl)"=w212) -> ()  [unwired: 2 in, 2 out]
                n138 = property on="SYS|Plot|Units" class="Arr (strict)"("Val(Sgnl)"=w211) -> ()  [unwired: 2 in, 2 out]
              }
            }
          }
          event "SYS|Plot|Names", "SYS|Plot|Units": Value Change {
            w214 = 100 ("dimension size")
            n139 = event-data() -> ()  [unwired: 1 in, 6 out]
            n140 = local read "SYS|Plot|Values"() -> (w223:sgl[])
            n141 = Not A Number/Path/Refnum?(number/path/refnum=w223) -> (NaN/Path/Refnum?=w222:bool[])
            n142 = for {
              tunnel: w223 -> [w226] mode=indexing
              tunnel: w222 -> [w227] mode=indexing
              tunnel: [w225] -> w216 mode=indexing
              n143 = case shown="False" w227 {
                tunnel: w226 -> [w228 _]
                tunnel: [w229 ""] -> w225
                frame False {
                  n144 = Format Into String(format string="%#_4p", w228) -> (resulting string=w229:string)  [unwired: 2 in, 1 out]
                }
                frame True {
                }
              }
            }
            n145 = local read "SYS|Plot|Names"() -> (w219:string[])
            n146 = local read "SYS|Plot|Units"() -> (w218:string[])
            n147 = Reshape Array(w219, w214) -> (w221:string[])
            n148 = Reshape Array(w218, w214) -> (w220:string[])
            n149 = Reshape Array(w216, w214) -> (w215:string[])
            n150 = Build Array(w221, w215, w220) -> (w224:string[][])
            n151 = Transpose 2D Array(2D array=w224) -> (transposed array=w217:string[][])
            n152 = property on="_QuickValues" class="MCListbox (strict)"("ItemNames"=w217) -> ()  [unwired: 2 in, 2 out]
          }
          event "_RedrawList": Value Change {
            n153 = event-data() -> ()  [unwired: 1 in, 1 out]
            n154 = local read "_Subhost-FP.DockStates"() -> (w237:bool[])
            n155 = local write "_RedrawList"(FALSE ("Redraw")) -> ()
            n156 = for {
              tunnel: w240 -> [w250] mode=indexing
              tunnel: [w249] -> w238 mode=indexing
              tunnel: w237 -> [w247] mode=indexing
              tunnel: [w243] -> w236 mode=indexing
              tunnel: [w242] -> w235 mode=indexing
              tunnel: w233 -> [w241]
              tunnel: [w241] -> w232
              i -> [w248]
              n157 = property class="VI"(reference=w250) -> ("FP.State"=w249:T10)  [unwired: 1 in, 2 out]
              n158 = case shown="\"Standard\", \"Minimized\", \"Maximized\"" w249 {
                tunnel: [FALSE TRUE] -> w246
                frame "Invalid", "Closed", "Hidden", Default {
                }
                frame "Standard", "Minimized", "Maximized" {
                }
              }
              n159 = Compound Arithmetic op=AND(w246, w247) -> (w243:bool)
              n160 = property on="_SubHost-List" class="LstBox (strict)"("Active Row"=w248, "CellFontBold"=w246) -> ()  [unwired: 2 in, 2 out]
              n161 = Select(t=16 ("Item Symbols"), s=w243, f=0 ("Item Symbols")) -> (s? t:f=w242:i32)
            }
            n162 = property on="_SubHost-List" class="LstBox (strict)"("Item Symbols"=w235) -> ()  [unwired: 2 in, 2 out]
            n163 = local write "_Subhost-FP.DockStates"(w236) -> ()
            n164 = local write "_Subhost-FP.States"(w238) -> ()
            n165 = call <vilib>:"Unset Busy.vi"("error in (no error)"=w232) -> ("error out"=w234:errorcluster)  [unwired: 10 in]
          }
          event "_SubHost-List": Value Change {
            n166 = event-data() -> ("NewVal"=w253:i32)  [unwired: 1 in]
            n167 = local read "_Subhost-FP.DockStates"() -> (w259:bool[])
            n168 = call <vilib>:"Set Busy.vi"("error in (no error)"=w255) -> ("error out"=w257:errorcluster)  [unwired: 9 in, 1 out]
            n169 = property on="_RedrawList" class="Bool (strict)"(error in=w257, "Val(Sgnl)"=TRUE ("Value (Signaling)")) -> (error out=w256:errorcluster)  [unwired: 1 in, 1 out]
            n170 = case shown="0, Default" w253 {
              selector: w253 -> [_ w266]
              tunnel: w258 -> [_ w268]
              tunnel: w259 -> [_ w267]
              tunnel: w256 -> [w261 w263]
              tunnel: [w261 w262] -> w254
              frame -1 {
              }
              frame 0, Default {
                n171 = Index Array(array=w267, index=w266) -> (element=w265:bool)
                n172 = Index Array(array=w268, index=w266) -> (element=w269:refnum<vi>)
                n173 = case shown="False" w265 {
                  tunnel: w269 -> [w277 w321]
                  tunnel: w263 -> [w272 w320]
                  tunnel: [w271 w319] -> w262
                  frame False {
                    n174 = global read "VI Ref Global.vi" "PanelRef"() -> (w273:refnum<vi>)
                    n175 = property class="VI"(reference=w277, error in=w272) -> (reference out=w275:refnum<vi>, error out=w274:errorcluster, "FP.State"=w276:T10)
                    n176 = property on="_AutoFit" class="Bool (strict)"("Val(Sgnl)"=TRUE ("Value (Signaling)")) -> ()  [unwired: 2 in, 2 out]
                    n177 = case shown="\"Standard\", Default" w276 {
                      tunnel: w275 -> [_ w303]
                      tunnel: w274 -> [w280 w299]
                      tunnel: w273 -> [w283 w302]
                      tunnel: [w281 w300] -> w271
                      frame "Standard", Default {
                        n178 = invoke on="_DisplayPanel" class="SubPnl" method="Remove VI"(error in=w280) -> (error out=w279:errorcluster)  [unwired: 2 in, 2 out]
                        n179 = Not A Number/Path/Refnum?(number/path/refnum=w283) -> (NaN/Path/Refnum?=w282:bool)
                        n180 = case shown="False" w282 {
                          tunnel: w283 -> [w288 _]
                          tunnel: w279 -> [w287 w296]
                          tunnel: [w285 w296] -> w281
                          frame False {
                            n181 = property class="VI"(reference=w288, error in=w287) -> (reference out=w289:refnum<vi>, error out=w286:errorcluster, "FP.State"=w284:T10)
                            n182 = case shown="\"Hidden\", Default" w284 {
                              tunnel: w289 -> [_ w295]
                              tunnel: w286 -> [w290 w292]
                              tunnel: [w290 w291] -> w285
                              frame "Hidden", Default {
                              }
                              frame "Closed" {
                                n183 = invoke class="VI" method="FP.Open"(reference=w295, error in=w292, "Activate"=FALSE ("Activate?"), "State"=T10."Hidden") -> (error out=w291:errorcluster)  [unwired: 1 in, 4 out]
                              }
                            }
                          }
                          frame True {
                          }
                        }
                        n184 = global write "VI Ref Global.vi" "PanelRef"(refnum<vi> refnum ("PanelRef")) -> ()
                      }
                      frame "Hidden" {
                        n185 = invoke on="_DisplayPanel" class="SubPnl" method="Remove VI"(error in=w299) -> (error out=w298:errorcluster)  [unwired: 2 in, 2 out]
                        n186 = Not A Number/Path/Refnum?(number/path/refnum=w302) -> (NaN/Path/Refnum?=w301:bool)
                        n187 = case shown="False" w301 {
                          tunnel: [w311 w318] -> w305
                          tunnel: w298 -> [w309 w318]
                          tunnel: w302 -> [w308 _]
                          frame False {
                            n188 = property class="VI"(reference=w308, error in=w309) -> (reference out=w307:refnum<vi>, error out=w310:errorcluster, "FP.State"=w306:T10)
                            n189 = case shown="\"Closed\"" w306 {
                              tunnel: w307 -> [_ w317]
                              tunnel: w310 -> [w312 w314]
                              tunnel: [w312 w313] -> w311
                              frame "Hidden", Default {
                              }
                              frame "Closed" {
                                n190 = invoke class="VI" method="FP.Open"(reference=w317, error in=w314, "Activate"=FALSE ("Activate?"), "State"=T10."Hidden") -> (error out=w313:errorcluster)  [unwired: 1 in, 4 out]
                              }
                            }
                          }
                          frame True {
                          }
                        }
                        n191 = invoke class="VI" method="FP.Close"(reference=w303, error in=w305) -> (reference out=w297:refnum<vi>, error out=w304:errorcluster)  [unwired: 1 in, 1 out]
                        n192 = invoke on="_Panel" class="SubPnl" method="Insert VI"(error in=w304, "VI Ref"=w297) -> (error out=w300:errorcluster)  [unwired: 2 in, 3 out]
                        n193 = global write "VI Ref Global.vi" "PanelRef"(w297) -> ()
                      }
                    }
                  }
                  frame True {
                    n194 = property class="VI"(reference=w321, error in=w320) -> (reference out=w323:refnum<vi>, error out=w322:errorcluster, "FP.State"=w324:T10)
                    n195 = case shown="\"Invalid\", \"Closed\", \"Hidden\"" w324 {
                      selector: w324 -> [w328 _]
                      tunnel: w323 -> [w329 _]
                      tunnel: w322 -> [w327 w330]
                      tunnel: [w326 w330] -> w319
                      frame "Standard", "Minimized", "Maximized", Default {
                        n196 = invoke class="VI" method="FP.Open"(reference=w329, error in=w327, "Activate"=TRUE ("Activate?"), "State"=w328) -> (error out=w326:errorcluster)  [unwired: 1 in, 4 out]
                      }
                      frame "Invalid", "Closed", "Hidden" {
                      }
                    }
                  }
                }
                n197 = local write "_SubHost-List"(-1 ("_SubHost-List")) -> ()
              }
            }
          }
          event "_SubHost-List": Shortcut Menu Activation? {
            w353 = 12  # Header Height
            n198 = event-data() -> ("Coords.Vertical"=w345:i32, "CtlRef"=w346:refnum<vi>, "MenuRef"=w356:refnum<k9>)  [unwired: 1 in]
            n199 = property on="Property Node" class="LstBox (strict)"(reference=w346) -> ("Top"=w352:i32, "Cell Height"=w350:i32, "Top Row"=w347:i32)  [unwired: 1 in, 2 out]
            n200 = local read "_Subhost-FP.DockStates"() -> (w344:bool[])
            n201 = Increment(x=w350) -> (x+1=w348:i32)
            n202 = Compound Arithmetic op=ADD(invert w353, w345, invert w352) -> (w351:i32)
            n203 = Quotient & Remainder(x=w351, y=w348) -> (floor(x/y)=w349:i32)  [unwired: 1 out]
            n204 = Add(x=w349, y=w347) -> (x+y=w333:i32)
            n205 = Index Array(array=w344, index=w333) -> (element=w339:bool)
            n206 = Index Array(array=w334, index=w333) -> (element=w331:refnum<vi>)
            n207 = Not A Number/Path/Refnum?(number/path/refnum=w331) -> (NaN/Path/Refnum?=w332:bool)
            n208 = Delete Menu Items(6:w336, 9:w356) -> (0:w354:errorcluster, 3:w355:refnum<k9>)  [unwired: 2 in]
            n209 = Select(t="Dock" ("item names"), s=w339, f="Undock" ("item names")) -> (s? t:f=w337:string)
            n210 = Select(t="_DOCK" ("format string"), s=w339, f="_UNDOCK" ("format string")) -> (s? t:f=w338:string)
            n211 = case shown="False" w332 {
              tunnel: w355 -> [w361 _]
              tunnel: w354 -> [w360 w362]
              tunnel: w338 -> [w359 _]
              tunnel: w337 -> [w358 _]
              tunnel: [w357 w362] -> w335
              frame False {
                n212 = Insert Menu Items(6:w360, 7:w359, 8:w358, 9:w361) -> (0:w357:errorcluster)  [unwired: 2 in, 2 out]
              }
              frame True {
              }
            }
            n213 = event-data() -> ()  [unwired: 2 in, 1 out]
          }
          event "_SubHost-List": Shortcut Menu Selection (User) {
            w380 = 12  # Header Height
            n214 = event-data() -> ("Coords.Vertical"=w372:i32, "CtlRef"=w373:refnum<vi>, "ItemTag"=w371:string)  [unwired: 1 in]
            n215 = call <vilib>:"Set Busy.vi"("error in (no error)"=w365) -> ("error out"=w364:errorcluster)  [unwired: 9 in, 1 out]
            n216 = property on="Property Node" class="LstBox (strict)"(reference=w373) -> ("Top"=w379:i32, "Cell Height"=w377:i32, "Top Row"=w374:i32)  [unwired: 1 in, 2 out]
            n217 = property on="_RedrawList" class="Bool (strict)"(error in=w364, "Val(Sgnl)"=TRUE ("Value (Signaling)")) -> (error out=w366:errorcluster)  [unwired: 1 in, 1 out]
            n218 = global read "VI Ref Global.vi" "PanelRef"() -> (w363:refnum<vi>)
            n219 = Increment(x=w377) -> (x+1=w375:i32)
            n220 = Compound Arithmetic op=ADD(invert w380, w372, invert w379) -> (w378:i32)
            n221 = Quotient & Remainder(x=w378, y=w375) -> (floor(x/y)=w376:i32)  [unwired: 1 out]
            n222 = Add(x=w376, y=w374) -> (x+y=w368:i32)
            n223 = case shown="\"_UNDOCK\"" w371 {
              tunnel: w370 -> [w396 _ w422]
              tunnel: w368 -> [w395 _ w421]
              tunnel: w363 -> [w381 _ w420]
              tunnel: [w387 w410 w419] -> w367
              tunnel: w366 -> [w388 w410 w411]
              frame "_DOCK" {
                n224 = local read "_Subhost-FP.DockStates"() -> (w394:bool[])
                n225 = invoke on="_DisplayPanel" class="SubPnl" method="Remove VI"(error in=w388) -> (error out=w384:errorcluster)  [unwired: 2 in, 2 out]
                n226 = Index Array(array=w396, index=w395) -> (element=w383:refnum<vi>)
                n227 = Not A Number/Path/Refnum?(number/path/refnum=w381) -> (NaN/Path/Refnum?=w382:bool)
                n228 = case shown="False" w382 {
                  tunnel: w384 -> [w401 w409]
                  tunnel: [w399 w409] -> w385
                  tunnel: w381 -> [w397 _]
                  frame False {
                    n229 = property class="VI"(reference=w397, error in=w401) -> (reference out=w402:refnum<vi>, error out=w400:errorcluster, "FP.State"=w398:T10)
                    n230 = case shown="\"Closed\"" w398 {
                      tunnel: w402 -> [_ w408]
                      tunnel: w400 -> [w403 w405]
                      tunnel: [w403 w404] -> w399
                      frame "Hidden", Default {
                      }
                      frame "Closed" {
                        n231 = invoke class="VI" method="FP.Open"(reference=w408, error in=w405, "Activate"=FALSE ("Activate?"), "State"=T10."Hidden") -> (error out=w404:errorcluster)  [unwired: 1 in, 4 out]
                      }
                    }
                  }
                  frame True {
                  }
                }
                n232 = Replace Array Subset(array=w394, new element=FALSE ("new element/subarray"), index=w395) -> (w393:bool[])
                n233 = local write "_Subhost-FP.DockStates"(w393) -> ()
                n234 = invoke class="VI" method="FP.Close"(reference=w383, error in=w385) -> (reference out=w390:refnum<vi>, error out=w389:errorcluster)  [unwired: 1 in, 1 out]
                n235 = invoke on="_Panel" class="SubPnl" method="Insert VI"(error in=w389, "VI Ref"=w390) -> (error out=w386:errorcluster)  [unwired: 2 in, 3 out]
                n236 = global write "VI Ref Global.vi" "PanelRef"(w390) -> ()
                n237 = property on="_AutoFit" class="Bool (strict)"(error in=w386, "Val(Sgnl)"=TRUE ("Value (Signaling)")) -> (error out=w387:errorcluster)  [unwired: 1 in, 1 out]
              }
              frame Default {
              }
              frame "_UNDOCK" {
                n238 = Index Array(array=w422, index=w421) -> (element=w414:refnum<vi>)
                n239 = local read "_Subhost-FP.DockStates"() -> (w418:bool[])
                n240 = Equal?(x=w420, y=w414) -> (x = y?=w415:bool)
                n241 = case shown="True" w415 {
                  tunnel: w414 -> [w426 w431]
                  tunnel: w411 -> [w424 w429]
                  tunnel: [w423 w430] -> w412
                  frame False {
                    n242 = property class="VI"(reference=w426, error in=w424, "FP.State"=T10."Standard" ("Front Panel Window:State")) -> (error out=w423:errorcluster)  [unwired: 1 out]
                  }
                  frame True {
                    n243 = invoke on="_DisplayPanel" class="SubPnl" method="Remove VI"(error in=w429) -> (error out=w428:errorcluster)  [unwired: 2 in, 2 out]
                    n244 = global write "VI Ref Global.vi" "PanelRef"(refnum<vi> refnum ("PanelRef")) -> ()
                    n245 = invoke class="VI" method="FP.Open"(reference=w431, error in=w428, "Activate"=TRUE ("Activate?"), "State"=T10."Standard") -> (error out=w430:errorcluster)  [unwired: 1 in, 4 out]
                  }
                }
                n246 = Replace Array Subset(array=w418, new element=TRUE ("new element/subarray"), index=w421) -> (w417:bool[])
                n247 = local write "_Subhost-FP.DockStates"(w417) -> ()
                n248 = property on="_AutoFit" class="Bool (strict)"(error in=w412, "Val(Sgnl)"=TRUE ("Value (Signaling)")) -> (error out=w419:errorcluster)  [unwired: 1 in, 1 out]
              }
            }
          }
          event Key Down {
            n249 = event-data() -> ("PlatMods"=w434:T38, "VKey"=w439:T39, "FocusObj"=w438:refnum<vi>)  [unwired: 1 in]
            n250 = property class="GObj"(reference=w438) -> ("ClassID"=w437:u32)  [unwired: 1 in, 2 out]
            n251 = case shown="0, Default" w437 {
              tunnel: w439 -> [w441 w448]
              tunnel: [_ w447] -> w436
              tunnel: w435 -> [_ w446]
              tunnel: w434 -> [w442 _]
              frame 0, Default {
                n252 = Unbundle By Name(w442) -> ("Ctrl"=w440:bool)
                n253 = case shown="\"F2\"" w441 {
                  tunnel: w440 -> [_ w443]
                  frame "ASCII", Default {
                  }
                  frame "F2" {
                    n254 = case shown="False" w443 {
                      frame False {
                      }
                      frame True {
                        n255 = vi-ref "System-Hidden-Settings-Host.vi"() -> (w445:refnum<vi>)
                        n256 = property class="VI"(reference=w445, "FP.State"=T10."Standard" ("Front Panel Window:State")) -> ()  [unwired: 1 in, 2 out]
                      }
                    }
                  }
                }
              }
              frame 46 {
                n257 = case shown="\"Delete\"" w448 {
                  tunnel: [_ w449] -> w447
                  tunnel: w446 -> [_ w449]
                  frame "ASCII", Default {
                  }
                  frame "Delete" {
                    w455 = "" ("Units")
                    w456 = 100 ("dimension size")
                    n258 = property on="SYS|Plot|Names" class="Arr (strict)"() -> ("Value"=w461:string[])  [unwired: 2 in, 2 out]
                    n259 = property on="SYS|Plot|Units" class="Arr (strict)"() -> ("Value"=w462:string[])  [unwired: 2 in, 2 out]
                    n260 = property on="SYS|Plot|IDs" class="Arr (strict)"() -> ("Value"=w460:T2)  [unwired: 2 in, 2 out]
                    n261 = local read "_QuickValues"() -> (w450:i32)
                    n262 = Reshape Array(w461, w456) -> (w457:string[])
                    n263 = Reshape Array(w462, w456) -> (w458:string[])
                    n264 = Reshape Array(w460, w456) -> (w459:T2)
                    n265 = Replace Array Subset(array=w457, new element=w455, index=w450) -> (w453:string[])
                    n266 = Replace Array Subset(array=w458, new element=w455, index=w450) -> (w452:string[])
                    n267 = Replace Array Subset(array=w459, new element=T3 {"ID"=0, "Element"=[]} ("ID"), index=w450) -> (w451:T2)
                    n268 = property on="SYS|Plot|Names" class="Arr (strict)"("Val(Sgnl)"=w453) -> ()  [unwired: 2 in, 2 out]
                    n269 = property on="SYS|Plot|Units" class="Arr (strict)"("Val(Sgnl)"=w452) -> ()  [unwired: 2 in, 2 out]
                    n270 = property on="SYS|Plot|IDs" class="Arr (strict)"("Val(Sgnl)"=w451) -> ()  [unwired: 2 in, 2 out]
                  }
                }
              }
            }
          }
          event "SYS|Host|Fault": Mouse Down {
            n271 = event-data() -> ()  [unwired: 1 in, 8 out]
            n272 = call <vilib>:"SCM Console Button.vi"("Button"=T11."Fault Display") -> ()
          }
          event "_CalScope": Value Change {
            n273 = event-data() -> ()  [unwired: 1 in, 6 out]
            n274 = local write "_CalScope"(FALSE ("_CalScope")) -> ()
            n275 = call <vilib>:"SCM Console Button.vi"("Button"=T11."CalScope") -> ()
          }
          event "_CalTrend": Value Change {
            n276 = event-data() -> ()  [unwired: 1 in, 6 out]
            n277 = local write "_CalTrend"(FALSE ("_CalScope")) -> ()
            n278 = call <vilib>:"SCM Console Button.vi"("Button"=T11."CalTrend") -> ()
          }
          event "_CalSave": Value Change {
            n279 = event-data() -> ()  [unwired: 1 in, 6 out]
            n280 = local write "_CalSave"(FALSE ("_CalScope")) -> ()
            n281 = call <vilib>:"SCM Console Button.vi"("Button"=T11."Save Calibration") -> ()
          }
          event "_CalSaveAs": Value Change {
            n282 = event-data() -> ()  [unwired: 1 in, 6 out]
            n283 = local write "_CalSaveAs"(FALSE ("_CalScope")) -> ()
            n284 = call <vilib>:"SCM Console Button.vi"("Button"=T11."Save Calibration As") -> ()
          }
          event "_CalLoad": Value Change {
            n285 = event-data() -> ()  [unwired: 1 in, 6 out]
            n286 = local write "_CalLoad"(FALSE ("_CalScope")) -> ()
            n287 = call <vilib>:"SCM Console Button.vi"("Button"=T11."Load Calibration File") -> ()
          }
          event "_AutoFit": Value Change {
            n288 = event-data() -> ()  [unwired: 1 in, 1 out]
            n289 = property on="_DisplayPanel" class="SubPnl"() -> (error out=w485:errorcluster, "InsertedVI"=w481:refnum<vi>)  [unwired: 2 in, 1 out]
            n290 = local write "_AutoFit"(FALSE ("_Fit")) -> ()
            n291 = Not A Number/Path/Refnum?(number/path/refnum=w481) -> (NaN/Path/Refnum?=w482:bool)
            n292 = case shown="False" w482 {
              tunnel: w480 -> [w529 _]
              tunnel: w481 -> [w528 _]
              tunnel: w485 -> [w508 _]
              tunnel: w484 -> [w506 w542]
              tunnel: [w499 w540] -> w483
              frame False {
                n293 = property class="VI"(reference=w529, error in=w506) -> (error out=w505:errorcluster, "Panel"=w530:refnum<vi>)  [unwired: 1 out]
                n294 = property class="VI"(reference=w528, error in=w508) -> (error out=w491:errorcluster, "Minimum Panel Size"=w507:T40, "Panel"=w498:refnum<vi>)  [unwired: 1 out]
                n295 = property class="Pnl"(reference=w530, error in=w505, "DeferPanUpdts"=TRUE ("Defer Panel Updates")) -> (reference out=w493:refnum<vi>, "Bounds"=w515:T8)  [unwired: 1 out]
                n296 = property on="Top left icons" class="Pane"() -> ("Height"=w521:u32)  [unwired: 2 in, 2 out]
                n297 = property on="Splitter 4" class="Splitter"() -> ("Height"=w520:u32)  [unwired: 2 in, 2 out]
                n298 = property on="Indicators" class="Pane"() -> ("Height"=w519:u32)  [unwired: 2 in, 2 out]
                n299 = property on="Splitter" class="Splitter"() -> ("Height"=w518:u32)  [unwired: 2 in, 2 out]
                n300 = property on="Subhosts" class="Pane"() -> ("Width"=w526:u32)  [unwired: 2 in, 2 out]
                n301 = property on="Splitter 2" class="Splitter"() -> ("Width"=w525:u32)  [unwired: 2 in, 2 out]
                n302 = property on="Quickvalues" class="Pane"() -> ("Width"=w524:u32)  [unwired: 2 in, 2 out]
                n303 = property on="Splitter 3" class="Splitter"() -> ("Width"=w523:u32)  [unwired: 2 in, 2 out]
                n304 = property class="Pnl"(reference=w498, error in=w491, "DeferPanUpdts"=TRUE ("Defer Panel Updates")) -> (reference out=w492:refnum<vi>, error out=w490:errorcluster)
                n305 = Unbundle(w515) -> ("Width"=w527:u32, "Height"=w522:u32)
                n306 = Compound Arithmetic op=ADD(w527, invert w526, invert w525, invert w524, invert w523) -> (w517:u32)
                n307 = Compound Arithmetic op=ADD(w522, invert w521, invert w520, invert w519, invert w518) -> (w516:u32)
                n308 = Bundle(cluster=w515, "Width"=w517, "Height"=w516) -> (w510:T8)
                n309 = invoke on="_DisplayPanel" class="SubPnl" method="FitControlToPane"(error in=w490) -> (error out=w489:errorcluster)  [unwired: 2 in, 2 out]
                n310 = Unbundle(w507) -> ("Horizontal"=w514:i16, "Vertical"=w512:i16)
                n311 = Unbundle(w510) -> ("Width"=w513:u32, "Height"=w511:u32)
                n312 = Less?(x=w514, y=w513) -> (x < y?=w503:bool)
                n313 = Less?(x=w512, y=w511) -> (x < y?=w504:bool)
                n314 = And(x=w503, y=w504) -> (x .and. y?=w509:bool)
                n315 = case shown="False" w509 {
                  tunnel: w507 -> [w534 _]
                  tunnel: w489 -> [w531 w539]
                  tunnel: [w531 w539] -> w500
                  tunnel: w504 -> [w536 _]
                  tunnel: w503 -> [w535 _]
                  frame False {
                    n316 = Unbundle(w534) -> ("Horizontal"=w533:i16, "Vertical"=w532:i16)
                    n317 = case shown="False" w535 {
                      tunnel: w533 -> [w538 _]
                      frame False {
                        n318 = property on="_DisplayPanel" class="SubPnl"("Width"=w538) -> ()  [unwired: 2 in, 2 out]
                      }
                      frame True {
                      }
                    }
                    n319 = case shown="False" w536 {
                      tunnel: w532 -> [w537 _]
                      frame False {
                        n320 = property on="_DisplayPanel" class="SubPnl"("Height"=w537) -> ()  [unwired: 2 in, 2 out]
                      }
                      frame True {
                      }
                    }
                  }
                  frame True {
                  }
                }
                n321 = Boolean To (0,1)(Boolean=w503) -> (0, 1=w488:i16)
                n322 = Boolean To (0,1)(Boolean=w504) -> (0, 1=w487:i16)
                n323 = property on="Subpanel" class="Pane"(error in=w500, "HorizScrollbarVisibility"=w488, "VertScrollbarVisibility"=w487) -> (error out=w494:errorcluster)  [unwired: 1 in, 1 out]
                n324 = property class="Pnl"(reference=w492, error in=w494, "DeferPanUpdts"=FALSE ("Defer Panel Updates")) -> (error out=w495:errorcluster)  [unwired: 1 out]
                n325 = property class="Pnl"(reference=w493, error in=w495, "DeferPanUpdts"=FALSE ("Defer Panel Updates")) -> (error out=w499:errorcluster)  [unwired: 1 out]
              }
              frame True {
                w543 = T41."Always Off" ("Horizontal Scrollbar Visibility")
                n326 = invoke on="_DisplayPanel" class="SubPnl" method="FitControlToPane"(error in=w542) -> (error out=w541:errorcluster)  [unwired: 2 in, 2 out]
                n327 = property on="Subpanel" class="Pane"(error in=w541, "HorizScrollbarVisibility"=w543, "VertScrollbarVisibility"=w543) -> (error out=w540:errorcluster)  [unwired: 1 in, 1 out]
              }
            }
          }
          event "_Help": Value Change {
            n328 = event-data() -> ()  [unwired: 1 in, 6 out]
            n329 = local write "_Help"(FALSE ("_Help")) -> ()
            n330 = Current VI's Path() -> (path=w548:path)
            n331 = Strip Path(path=w548) -> (stripped path=w547:path)  [unwired: 1 out]
            n332 = Build Path(base path=w547, name or relative path="DCM DSI User Guide.pdf") -> (appended path=w545:path)
            n333 = call <vilib>:"Open a Document on Disk.vi"("document path"=w545) -> ("error out"=w544:errorcluster)  [unwired: 6 in]
            n334 = case shown="Error" w544 {
              frame No Error {
              }
              frame Error {
                n335 = One Button Dialog(message="Help file missing") -> ()  [unwired: 1 in, 1 out]
              }
            }
          }
          event Panel Close? {
            n336 = event-data() -> ()  [unwired: 1 in, 4 out]
            n337 = local read "_Subhost-FP.DockStates"() -> (w552:bool[])
            n338 = call "Workspace - Save.vi"("_Subhost-FP.DockStates"=w552, "This VI"=w554, "VI Refs"=w556, "Subhost Names"=w557) -> ("VI Refs out"=w555:refnum<vi>[])  [unwired: 5 in, 2 out]
            n339 = for {
              tunnel: w555 -> [w563] mode=indexing
              tunnel: [w560] -> w553
              n340 = property class="VI"(reference=w563, "FP.State"=T10."Hidden" ("Front Panel Window:State")) -> (reference out=w562:refnum<vi>)  [unwired: 1 in, 1 out]
              n341 = Close Reference(reference=w562) -> (error out=w560:errorcluster)  [unwired: 1 in]
            }
            n342 = flat-sequence {
              tunnel: w553 -> [_]
              frame #0 {
                n343 = call <vilib>:"SCM Console Button.vi"("Button"=T11."Stop Host Application") -> ()
              }
            }
            n344 = event-data("Discard?"=TRUE) -> ()  [unwired: 1 in, 1 out]
          }
        }
      }
      n345 = while {
        stop <- FALSE ("status") stop-if-true
        n346 = control-ref of="_QuickValues"() -> (w113:refnum<vi>)
        n347 = control-ref of="SYS|Plot|Names"() -> (w112:refnum<vi>)
        n348 = control-ref of="SYS|Plot|Units"() -> (w115:refnum<vi>)
        n349 = control-ref of="SYS|Plot|IDs"() -> (w114:refnum<vi>)
        n350 = call "CalpointMenu.vi"("SYS|Plot|IDs"=w114, "SYS|Plot|Units"=w115, "SYS|Plot|Names"=w112, "_QuickValues"=w113) -> ()  [unwired: 8 in]
      }
    }
  }
